vi "CreatePublicEvents.vi"(8 "error in (no error)":errorcluster, 11 "SystemController":refnum<class "SystemController.lvclass">) -> (0 "error out":errorcluster, 3 "SystemController out":refnum<class "SystemController.lvclass">)   [LabVIEW 2017, in "SystemController.lvclass"]
doc: "---------------------------------------------------------------\nJKI State Machine Objects™\nhttp://jki.net/state-machine-objects/\nCopyright (C) 2005-2015, JKI <info@jki.net>\nALL RIGHTS RESERVEDJKI State Machine Objects (SMO) 1.0.0.4\nJKI - JKI\nCopyright (c) 2015, JKI"
uses:
  SystemController.lvclass
  SystemController.lvclass/SystemController.ctl
  Typedefs/PublicEvents--SystemController.UIClosed.ctl
  <vilib>/JKI/JKI SMO/SMO/SMO.lvclass
panel:
  # "For instructions on how to use the JKI State Machine Objects, examples and video tutorials, visit:\nhttp://jki.net/state-machine-objects/\n\nJKI State Machine Objects™\nhttp://jki.net/state-machine-objects/\nCopyright (C) 2005-2015, JKI <info@jki.net>\nALL RIGHTS RESERVED"
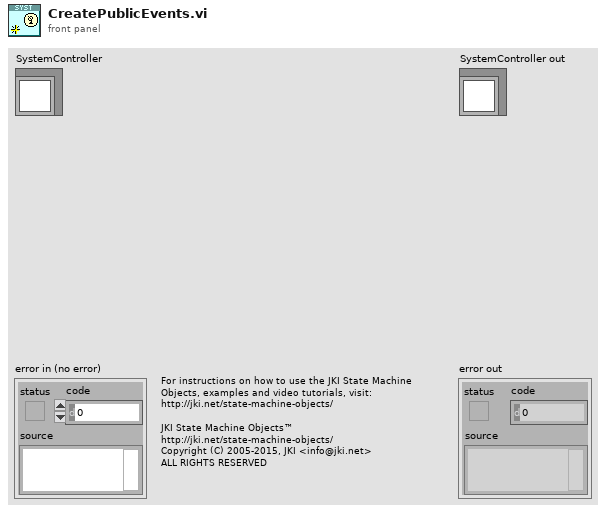
[diagram p1: front panel]
types:
  T1 = typedef "SystemController.lvclass/PrivateData--Ref.ctl" = refnum<data-value>
  T2 = typedef "SystemController.lvclass/PublicEvents--SystemController.UIClosed.ctl" = bool
  T3 = typedef "SystemController.lvclass/PrivateData--Cluster.ctl" = cluster{"Configuration":T4, "Dependencies":T8, "ProcessedImage":T9, "Public Events":T10}
  T4 = typedef "SystemController.lvclass/Configuration--Cluster.ctl" = cluster{"Camera":T5, "Find Eyes":bool, "Acquisition Rate (ms)":i32}
  T5 = typedef "SystemController.lvclass/CameraConfig--Cluster.ctl" = cluster{"Simulate Camera":bool, "IMAQ Camera":T6, "Simulated Camera Image":path}
  T6 = typedef "Camera_IMAQdx.lvclass/Configuration--Cluster.ctl" = cluster{"Camera Interface Name":string, "Number of Buffers":u32, "Image Name":string, "Image Type":T7}
  T7 = typedef "Image Type" = u32
  T8 = typedef "SystemController.lvclass/Dependencies--Cluster.ctl" = cluster{"Camera":refnum<class "Camera.lvclass">, "ImageFacialDetection":refnum<class "ImageFacialDetection.lvclass">}
  T9 = typedef "IMAQ Image.ctl" = refnum<image>
  T10 = typedef "SystemController.lvclass/PublicEvents--Cluster.ctl" = cluster{"UIClosed":refnum<user-event>}
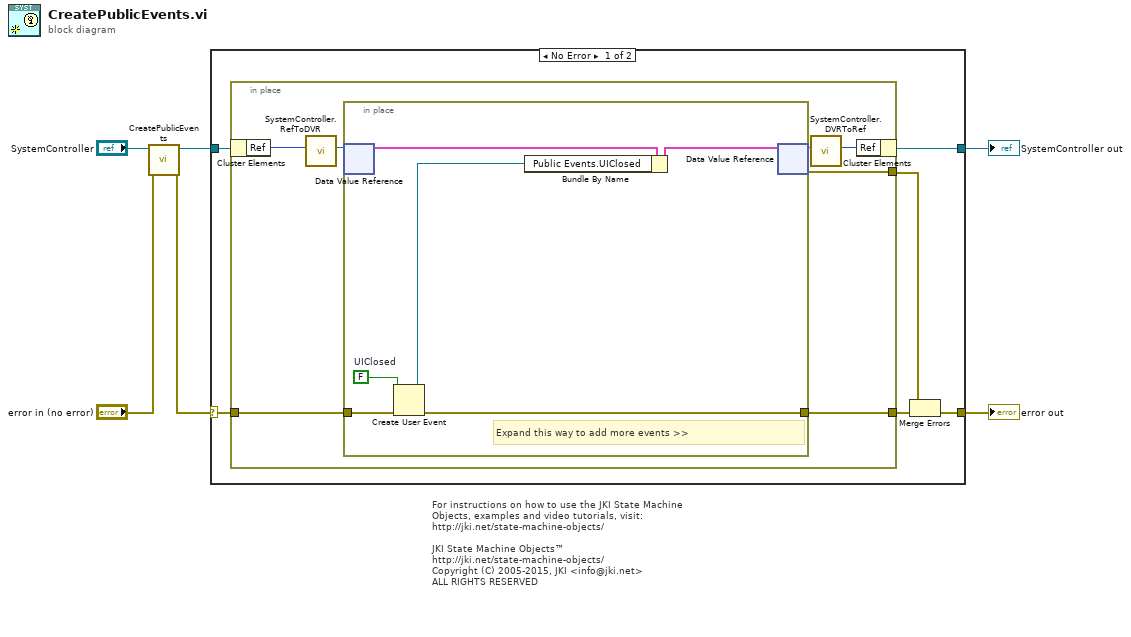
[diagram p0: block diagram]
diagram:
  # "For instructions on how to use the JKI State Machine Objects, examples and video tutorials, visit:\nhttp://jki.net/state-machine-objects/\n\nJKI State Machine Objects™\nhttp://jki.net/state-machine-objects/\nCopyright (C) 2005-2015, JKI <info@jki.net>\nALL RIGHTS RESERVED"
  n1 = call-parent "CreatePublicEvents.vi"("error in (no error)"="error in (no error)", "SMO"="SystemController") -> ("error out"=w1:errorcluster, "SMO out"=w3:refnum<class "SystemController.lvclass">)  [unwired: 8 in]
  n2 = case shown="No Error" w1 {
    selector: w1 -> [w10 w27]
    tunnel: [w8 w27] -> w5
    tunnel: [w11 w26] -> w6
    tunnel: w3 -> [w12 w26]
    frame No Error {
      n3 = in-place {
        in-place-border: w10 -> [w19]
        in-place-border: [w16] -> w7
        in-place-border: [w15] -> w9
        n4 = in-place-cluster #1(w12) -> ("Ref"=w18:u32)
        n5 = call "SystemController.RefToDVR.vi"("Ref"=w18) -> ("Ref"=w14:T1)  [unwired: 10 in]
        n6 = in-place {
          in-place-border: w19 -> [w25]
          in-place-border: [w22] -> w16
          w21 = T2 FALSE  # UIClosed
          # "Expand this way to add more events >>"
          n7 = in-place-dvr #2(w14) -> (w24:T3)  [unwired: 1 out]
          n8 = Create User Event(user event datatype=w21, error in=w25) -> (user event=w20:refnum<user-event>, error out=w22:errorcluster)
          n9 = Bundle By Name(cluster=w24, "Public Events.UIClosed"=w20) -> (w23:T3)
          n10 = in-place-dvr #2(w23) -> (w17:T1, w15:errorcluster)
        }
        n11 = call "SystemController.DVRToRef.vi"("Ref"=w17) -> ("Ref"=w13:u32)  [unwired: 10 in]
        n12 = in-place-cluster #1("Ref"=w13) -> (w11:refnum<class "SystemController.lvclass">)
      }
      n13 = Merge Errors(w9, w7) -> (w8:errorcluster)
    }
    frame Error {
    }
  }
  "error out" <- w5
  "SystemController out" <- w6
